vi "fixer.vi"(1 "2-10 flag":bool, 2 "input":T2) -> (0 "output":T1)   [LabVIEW 2013]
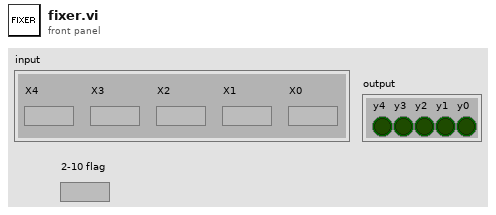
[diagram p1: front panel]
types:
  T1 = cluster{"y4":bool, "y3":bool, "y2":bool, "y1":bool, "y0":bool}
  T2 = cluster{"X4":bool, "X3":bool, "X2":bool, "X1":bool, "X0":bool}
  T3 = cluster{"Y5":bool, "Y4":bool, "Y3":bool, "Y2":bool, "Y1":bool, "Y0":bool}
  T4 = cluster{"Y4":bool, "Y3":bool, "Y2":bool, "Y1":bool, "Y0":bool}
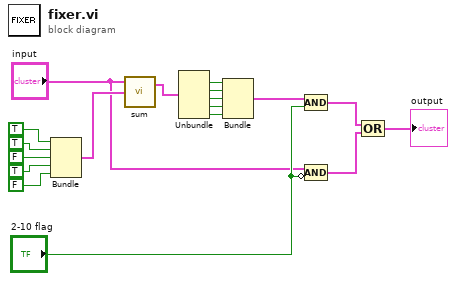
[diagram p0: block diagram]
diagram:
  n1 = Bundle(TRUE, TRUE, FALSE, TRUE, FALSE) -> (w13:cluster{bool, bool, bool, bool, bool})  [unwired: 1 in]
  n2 = call "sum.vi"("B"=w13, "A"="input") -> ("Output"=w12:T3)  [unwired: 1 in, 1 out]
  n3 = Unbundle(w12) -> ("Y4"=w7:bool, "Y3"=w8:bool, "Y2"=w9:bool, "Y1"=w10:bool, "Y0"=w11:bool)  [unwired: 1 out]
  n4 = Bundle("Y4"=w7, "Y3"=w8, "Y2"=w9, "Y1"=w10, "Y0"=w11) -> (w4:T4)  [unwired: 1 in]
  n5 = Compound Arithmetic op=AND(w4, "2-10 flag") -> (w3:T4)
  n6 = Compound Arithmetic op=AND("input", invert "2-10 flag") -> (w2:T2)
  n7 = Compound Arithmetic op=OR(w3, w2) -> (→"output":cluster{bool, bool, bool, bool, bool})
